vi "Turret Improved.vi"() -> ()   [LabVIEW 2016]
uses:
  <vilib>/Platform/TimedLoop/XDataNode/timing_clust.ctl
  <vilib>/Platform/TimedLoop/XDataNode/nitl_modes.ctl
  <vilib>/Platform/TimedLoop/XDataNode/wakeup.ctl
  TurretStates.ctl
  Drive Commands.ctl
  <vilib>/Analysis/coordinate.llb/Angle Units.ctl
  <vilib>/Analysis/coordinate.llb/Angle Range (Degree).ctl
  <vilib>/Analysis/coordinate.llb/Wrap Angle (scalar).vi
  <vilib>/platform/TimedLoop/XDataNode/XDataNode.xnode
  <vilib>/Platform/TimedLoop/XDataNode/XDNodeRunTimeDep.lvlib
  <vilib>/Analysis/NI_AAL_Angle.lvlib
panel:
  in  "Feed CW":dbl=0.02
  in  "FeedCCW":dbl=-0.02
  in  "Tab Control":T1(tab)
  in  "Min Rate":dbl=0.2
  in  "Lost Target Time?":dbl(knob)=0.5301133241962713 scale=0.0..1.0
  in  "Wait Time in Search":dbl(knob)=0.3769951386039123 scale=0.0..1.0
  in  "Period (ms)":dbl=100.0
  in  "Duty Cycle (%)":dbl=10.0
  in  "Target Range Gains":T2={"proportional gain (Kc)"=0.01, "integral time (Ti, min)"=0.005, "derivative time (Td, min)"=0.0} {"derivative time (Td, min)" format="%.4f"; "integral time (Ti, min)" format="%.8f"; "proportional gain (Kc)" format="%.8f"}
  in  "Target range":cluster{"output high":dbl, "output low":dbl}={"output high"=0.9, "output low"=-0.9}
  in  "Setpoint Tol":dbl=1.0
  in  "Search Gains":T2={"proportional gain (Kc)"=0.018, "integral time (Ti, min)"=0.003, "derivative time (Td, min)"=0.005}
  in  "Search Range":cluster{"output high":dbl, "output low":dbl}={"output high"=0.25, "output low"=-0.25}
  in  "Search Tol":dbl=10.0
  in  "Softstop":dbl=15.0
  in  "Jump to Desired Angle":T2={"proportional gain (Kc)"=0.0155, "integral time (Ti, min)"=0.003, "derivative time (Td, min)"=0.0}
  in  "Jump Output":cluster{"output high":dbl, "output low":dbl}={"output high"=0.5, "output low"=-0.5}
  in  "Valid Target Time Guess":dbl(knob)=0.19161068264500253 scale=0.0..1.0
  in  "Switch outer bound delta":dbl=20.0
  in  "Stable Movemt":dbl(knob)=0.11807450406305693 scale=0.0..1.0
  in  "Guess State Time?":u32
  out "TurretLate?":bool
  in  "Turret Max Speed":dbl(knob)=0.34982498966729664 scale=0.0..1.0
  in  "Reinitalize?":bool
  in  "Range for I":dbl=15.0
  out "Turret":cluster{"Double":dbl, "desired Angle":dbl}(graph)={"Double"=109.84640759396413, "desired Angle"=110.88007694880284}
  out "Motor Output":dbl=0.031700587068503525
  out "Turret State":dbl(graph)
  in  "Test LEDS":bool
  in  "CW Bound":dbl=130.0
  in  "CCW Bound":dbl=-90.0 format="%#_13g"
  in  "Turret Period":i64=20
  out "Turret Duration":i64
  out "Auto Target Lock":bool=TRUE
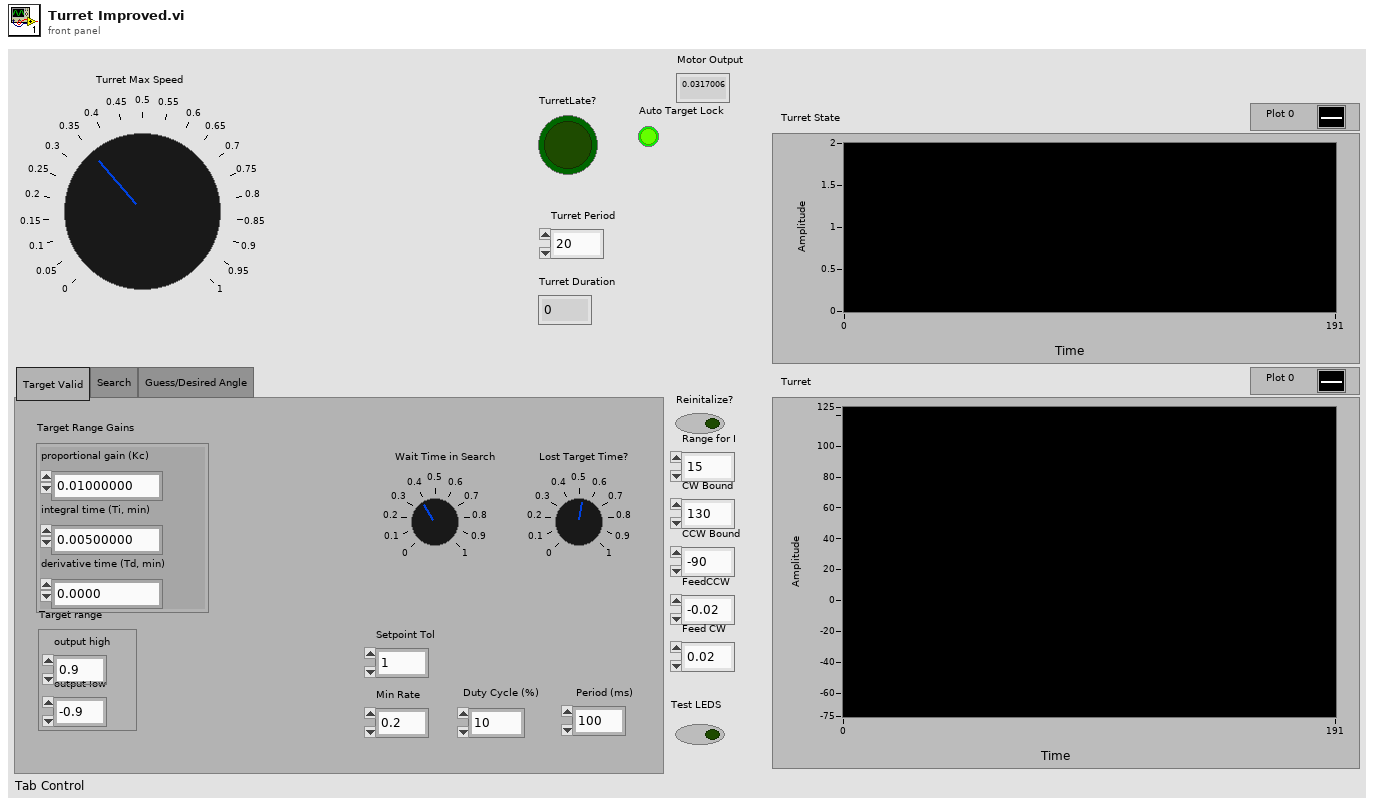
[diagram p1: front panel]
types:
  T1 = enum32{"Target Valid", "Search", "Guess/Desired Angle"}
  T2 = cluster{"proportional gain (Kc)":dbl, "integral time (Ti, min)":dbl, "derivative time (Td, min)":dbl}
  T3 = typedef "TurretStates.ctl" = enum16{"Target Valid in Range", "Guess", "Search", "Desired Angle Shot", "Manual"}
  T4 = typedef "XDNodeRunTimeDep.lvlib/timing_clust.ctl" = cluster{"Expected End [f-1]":u64, "Actual End [f-1]":u64, "Finished Late? [f-1]":bool, "Expected End [i-1]":u64, "Actual End [i-1]":u64, "Finished Late? [i-1]":bool, "Expected Start [i]":u64, "Actual Start [i]":u64, "Expected Start [f]":u64, "Actual Start [f]":u64, "Source Name":string, "Structure Name":string, "Period":i64, "Deadline":i64, "Offset":i64, "Start":i64, "Priority":i32, "Timeout":i32, "Mode":T5, "Wakeup Reason":T6, "Error":errorcluster, "Source Type":string, "Secondary Source Type":string, "Global End Time":u64, "Global Start Time":u64, "Frame Duration":u64, "Iteration Duration":u64, "Assigned CPU":i32, "I/O Scan Engine Mode":u32}
  T5 = typedef "XDNodeRunTimeDep.lvlib/nitl_modes.ctl" = enum32{"No Change", "Process missed periods, maintain original phase", "Discard missed periods, maintain original phase", "Process missed periods, ignore original phase", "Discard missed periods, ignore original phase"}
  T6 = typedef "XDNodeRunTimeDep.lvlib/wakeup.ctl" = enum32{"Normal", "Aborted", "Asynchronous wakeup", "Timing source error", "Timed loop error", "Timeout"}
  T7 = cluster{"Search Gains":cluster{"proportional gain (Kc)":dbl, "integral time (Ti, min)":dbl, "derivative time (Td, min)":dbl}, "Search Range":cluster{"output high":dbl, "output low":dbl}}
  T8 = cluster{"Jump to Desired Angle":cluster{"proportional gain (Kc)":dbl, "integral time (Ti, min)":dbl, "derivative time (Td, min)":dbl}, "Jump Output":cluster{"output high":dbl, "output low":dbl}}
  T9 = cluster{"Target Range Gains":cluster{"proportional gain (Kc)":dbl, "integral time (Ti, min)":dbl, "derivative time (Td, min)":dbl}, "Target range":cluster{"output high":dbl, "output low":dbl}}
  T10 = cluster{"Target Range Gains":cluster{"proportional gain (Kc)":dbl, "integral time (Ti, min)":dbl, "derivative time (Td, min)":dbl}, "Target range":cluster{"output high":dbl, "output low":dbl}}[]
  T11 = typedef "WPI_MotorControlDeviceRef.ctl" = cluster{"DeviceStatus":errorcluster, "Type":T12, "PWM":cluster{"PWM Channel":T13, "DeadBand":T14}, "CAN":cluster{"Device Number":u8, "SetOutput VI Ref":variant, "GetOutput VI Ref":variant, "Enable VI Ref":variant, "Disable VI Ref":variant, "Data":variant}, "Invert":bool}
  T12 = typedef "WPI_MotorControlType.ctl" = enum16{"PWM", "CAN"}
  T13 = typedef "FPGA_DIOPWMChannel.ctl" = enum8{"PWM 0", "PWM 1", "PWM 2", "PWM 3", "PWM 4", "PWM 5", "PWM 6", "PWM 7", "PWM 8", "PWM 9", "PWM MXP 0", "PWM MXP 1", "PWM MXP 2", "PWM MXP 3", "PWM MXP 4", "PWM MXP 5", "PWM MXP 6", "PWM MXP 7", "PWM MXP 8", "PWM MXP 9", "Invalid"}
  T14 = typedef "WPI_PWMDeadband.ctl" = cluster{"Name":string, "maxPositivePwm":i32, "minPositivePwm":i32, "centerPwm":i32, "maxNegativePwm":i32, "minNegativePwm":i32, "angularRange":u16}
  T15 = typedef "Drive Commands.ctl" = enum16{"Manual", "Get Gear", "Score Gear", "Align Rope", "Turn To Angle"}
  T16 = enum8{"setop", "setcolor", "default", "pilot", "ball", "gear", "both", "gearDeliver", "timeWarn", "targeting", "rave", "debug", "Set Power"}
  T17 = typedef "NI_AAL_Angle.lvlib/Angle Range (Degree).ctl" = u16
  T18 = typedef "NI_AAL_Angle.lvlib/Angle Units.ctl" = i32
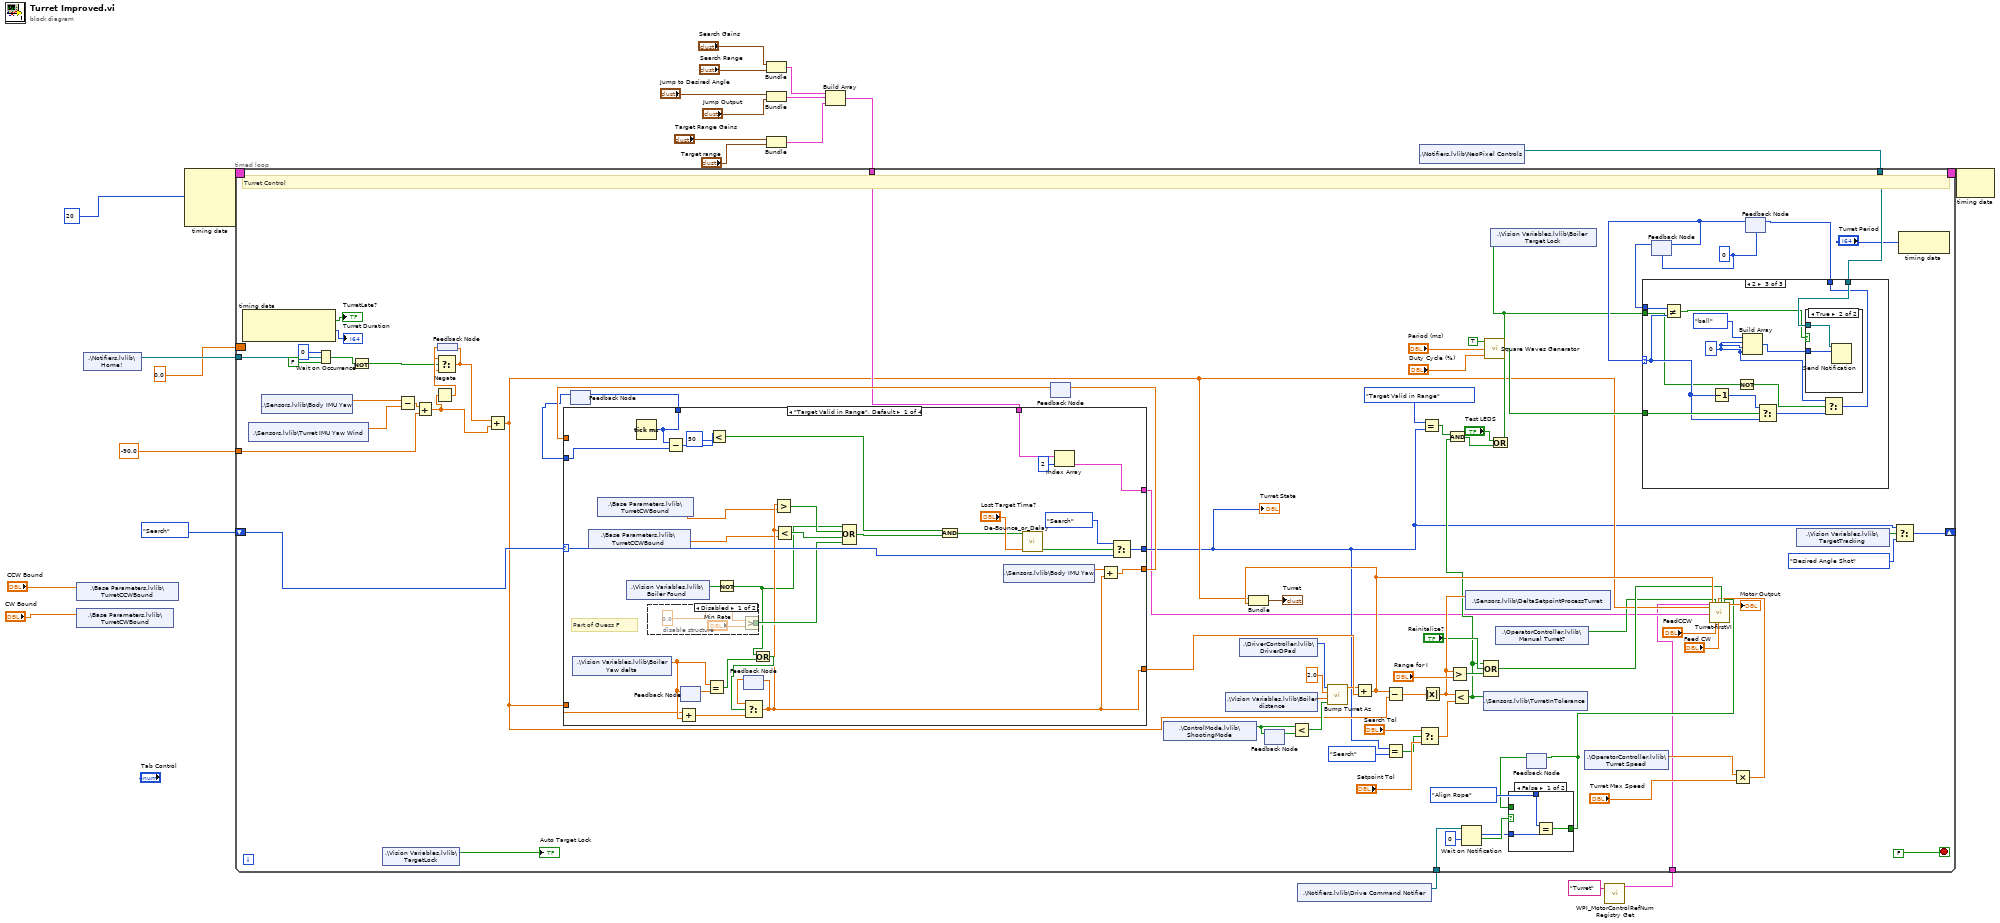
[diagram p0: block diagram]
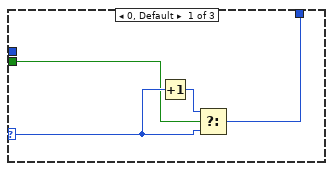
[diagram p3: hidden frame]
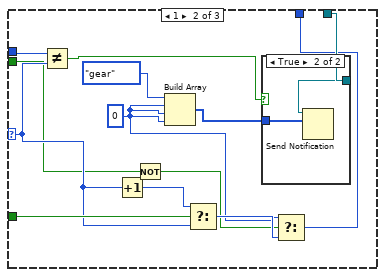
[diagram p4: hidden frame]
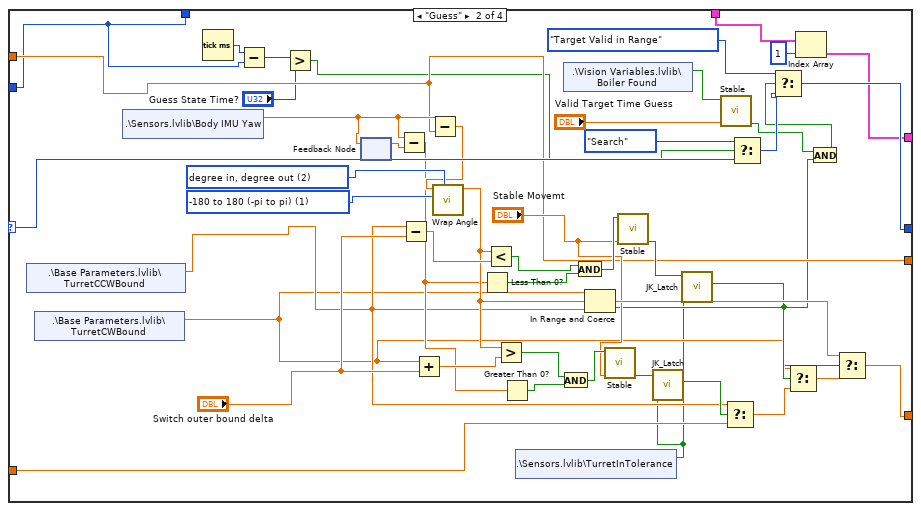
[diagram p8: hidden frame]
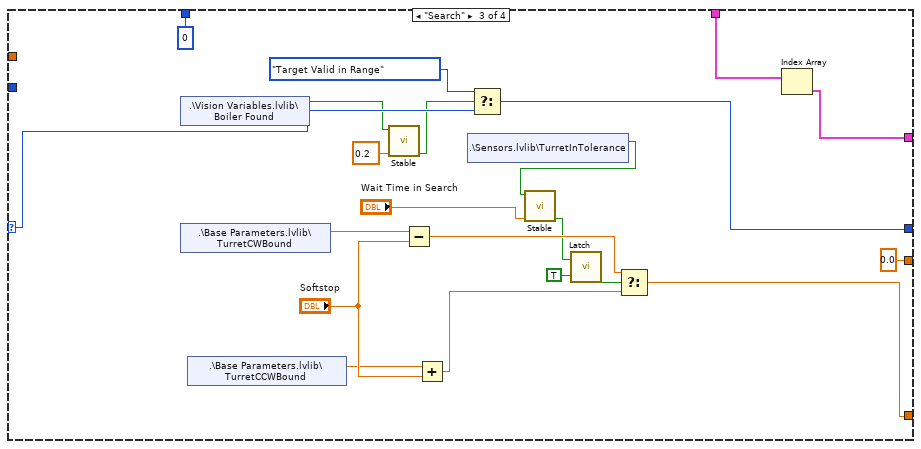
[diagram p9: hidden frame]
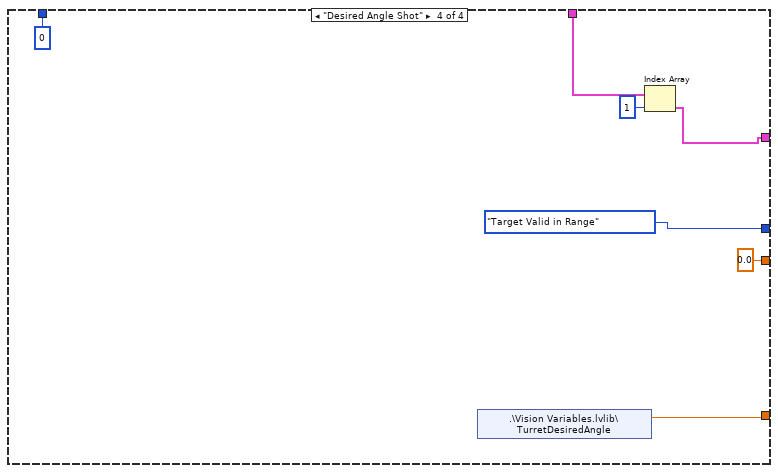
[diagram p10: hidden frame]
diagram:
  n1 = shared-variable ".\\Base Parameters.lvlib\\TurretCCWBound"("CCW Bound") -> ()  [unwired: 1 in, 1 out]
  n2 = shared-variable ".\\Base Parameters.lvlib\\TurretCWBound"("CW Bound") -> ()  [unwired: 1 in, 1 out]
  n3 = shared-variable ".\\Notifiers.lvlib\\Home!"() -> (w17:refnum<k4>)  [unwired: 1 in, 1 out]
  n4 = node-c288(i64 20 ("Period")) -> (w23:T4)  [unwired: 3 in]
  n5 = Bundle("Search Gains"="Search Gains", "Search Range"="Search Range") -> (w11:T7)  [unwired: 1 in]
  n6 = Bundle("Jump to Desired Angle"="Jump to Desired Angle", "Jump Output"="Jump Output") -> (w12:T8)  [unwired: 1 in]
  n7 = Bundle("Target Range Gains"="Target Range Gains", "Target range"="Target range") -> (w13:T9)  [unwired: 1 in]
  n8 = Build Array(w11, w12, w13) -> (w4:T10)
  n9 = shared-variable ".\\Notifiers.lvlib\\Drive Command Notifier"() -> (w3:refnum<notifier>)  [unwired: 1 in, 1 out]
  n10 = shared-variable ".\\Notifiers.lvlib\\NeoPixel Controls"() -> (w19:refnum<notifier>)  [unwired: 1 in, 1 out]
  n11 = call <vilib>:"WPI_MotorControlRefNum Registry Get.vi"("refnum name"="Turret") -> ("MotorControlDevRef"=w1:T11)  [unwired: 9 in, 1 out]
  n12 = timed-loop {
    timing: w23 -> [_]
    timing-out: [_] -> w22
    shift-right: [w58] -> _
    shift-left: TurretStates."Search" -> [w55]
    tunnel: w19 -> [w90]
    tunnel: -90.0 -> [w76]
    tunnel: w17 -> [w74]
    border: 0.0 -> [_]
    tunnel: w4 -> [w39]
    tunnel: w3 -> [w28]
    tunnel: w1 -> [w24]
    stop <- FALSE stop-if-true
    w83 = 0
    # "Turret Control"
    n13 = node-c288() -> (→"TurretLate?":bool, →"Turret Duration":i64)  [unwired: 1 in]
    n14 = shared-variable ".\\Sensors.lvlib\\Turret IMU Yaw Wind"() -> (w103:dbl)  [unwired: 1 in, 1 out]
    n15 = shared-variable ".\\Sensors.lvlib\\Body IMU Yaw"() -> (w102:dbl)  [unwired: 1 in, 1 out]
    n16 = Wait on Occurrence(1:FALSE ("ignore previous (T)"), 2:w74, 3:0 ("ms timeout (-1)")) -> (0:w72:bool)
    n17 = Not(x=w72) -> (.not. x?=w61:bool)
    n18 = shared-variable ".\\Vision Variables.lvlib\\TargetLock"() -> (→"Auto Target Lock":bool)  [unwired: 1 in, 1 out]
    n19 = Subtract(x=w102, y=w103) -> (x-y=w75:dbl)
    n20 = Add(x=w75, y=w76) -> (x+y=w63:dbl)
    n21 = Negate(x=w63) -> (-x=w65:dbl)
    n22 = feedback #1() -> (w64:dbl)
    n23 = Select(t=w65, s=w61, f=w64) -> (s? t:f=w62:dbl)
    n24 = feedback-in #1(w62) -> ()
    n25 = Add(x=w62, y=w63) -> (x+y=w36:dbl)
    n26 = feedback #2() -> (w92:u32)  [unwired: 1 in]
    n27 = feedback #3() -> (w97:dbl)  [unwired: 1 in]
    n28 = case shown="\"Target Valid in Range\", Default" w55 {
      selector: w55 -> [w169 w222 w243 _]
      tunnel: w36 -> [w164 w218 _ _]
      tunnel: [w148 w194 w245 TurretStates."Target Valid in Range"] -> w34
      tunnel: [w152 w215 w239 w250] -> w54
      tunnel: w97 -> [_ w196 _ _]
      tunnel: [w151 w196 0.0 ("Double") 0.0 ("Double")] -> w91
      tunnel: [w162 w187 u32 0 ("millisecond timer value") u32 0 ("millisecond timer value")] -> w93
      tunnel: w92 -> [w161 w187 _ _]
      tunnel: [w144 w178 w225 w247] -> w25
      tunnel: w39 -> [w143 w180 w226 w248]
      frame "Target Valid in Range", Default {
        # "Part of Guess F"
        n29 = shared-variable ".\\Vision Variables.lvlib\\Boiler Yaw delta"() -> (w173:dbl)  [unwired: 1 in, 1 out]
        n30 = shared-variable ".\\Base Parameters.lvlib\\TurretCCWBound"() -> (w147:dbl)  [unwired: 1 in, 1 out]
        n31 = shared-variable ".\\Base Parameters.lvlib\\TurretCWBound"() -> (w146:dbl)  [unwired: 1 in, 1 out]
        n32 = shared-variable ".\\Vision Variables.lvlib\\Boiler Found"() -> (w170:bool)  [unwired: 1 in, 1 out]
        n33 = Tick Count (ms)() -> (millisecond timer value=w162:u32)
        n34 = disable-structure shown="Disabled" {
          disable-tunnel: [w176 _] -> w163
          frame Disabled {
            n35 = Greater?(x=0.0, y="Min Rate") -> (0:w176:bool)
          }
          frame Enabled {
          }
        }
        n36 = Subtract(x=w162, y=w161) -> (x-y=w160:u32)
        n37 = Add(x=w164, y=w173) -> (x+y=w172:dbl)
        n38 = feedback-in #4(w173) -> ()
        n39 = feedback #4() -> (w174:dbl)  [unwired: 1 in]
        n40 = Equal?(x=w173, y=w174) -> (x = y?=w155:bool)
        n41 = Less?(x=w160, y=u32 50) -> (x < y?=w158:bool)
        n42 = Not(x=w170) -> (.not. x?=w150:bool)
        n43 = feedback #5() -> (w171:dbl)  [unwired: 1 in]
        n44 = Or(x=w150, y=w155) -> (x .or. y?=w154:bool)
        n45 = Select(t=w171, s=w154, f=w172) -> (s? t:f=w152:dbl)
        n46 = feedback-in #5(w152) -> ()
        n47 = Greater?(x=w152, y=w146) -> (0:w166:bool)
        n48 = Less?(x=w152, y=w147) -> (x < y?=w165:bool)
        n49 = Compound Arithmetic op=OR(w150, w166, w165, w163) -> (w157:bool)
        n50 = And(x=w158, y=w157) -> (x .and. y?=w156:bool)
        n51 = shared-variable ".\\Sensors.lvlib\\Body IMU Yaw"() -> (w153:dbl)  [unwired: 1 in, 1 out]
        n52 = call <userlib>:"De-Bounce_or_Delay.vi"("Eval Period (sec)"="Lost Target Time?", "Signal Input"=w156) -> ("Stable"=w149:bool)  [unwired: 9 in]
        n53 = Index Array(array=w143, index=2) -> (element=w144:T9)
        n54 = Add(x=w153, y=w152) -> (x+y=w151:dbl)
        n55 = Select(t=TurretStates."Search", s=w149, f=w169) -> (s? t:f=w148:T3)
      }
      frame "Guess" {
        w213 = T17 1 items=["none", "-180 to 180 (-pi to pi)", "0 to 360 (0 to 2pi)"] ("angle range")
        w214 = T18 2 items=["radian in, radian out", "radian in, degree out", "degree in, degree out", "degree in, radian out"] ("angle units")
        n56 = shared-variable ".\\Base Parameters.lvlib\\TurretCCWBound"() -> (w183:dbl)  [unwired: 1 in, 1 out]
        n57 = shared-variable ".\\Base Parameters.lvlib\\TurretCWBound"() -> (w182:dbl)  [unwired: 1 in, 1 out]
        n58 = shared-variable ".\\Sensors.lvlib\\Body IMU Yaw"() -> (w208:dbl)  [unwired: 1 in, 1 out]
        n59 = Tick Count (ms)() -> (millisecond timer value=w188:u32)
        n60 = Subtract(x=w188, y=w187) -> (x-y=w186:u32)
        n61 = Greater?(x=w186, y="Guess State Time?") -> (0:w184:bool)
        n62 = feedback-in #6(w208) -> ()
        n63 = feedback #6() -> (w209:dbl)  [unwired: 1 in]
        n64 = Subtract(x=w208, y=w209) -> (x-y=w202:dbl)
        n65 = Subtract(x=w183, y="Switch outer bound delta") -> (x-y=w220:dbl)
        n66 = Add(x=w182, y="Switch outer bound delta") -> (x+y=w219:dbl)
        n67 = Subtract(x=w208, y=w196) -> (x-y=w212:dbl)
        n68 = call-poly <vilib>:"Wrap Angle.vi"("angle units"=w214, "angle range"=w213, "angle in"=w212) -> ("angle out"=w211:dbl)  [unwired: 7 in, 1 out]
        n69 = Less Than 0?(x=w202) -> (x < 0?=w205:bool)
        n70 = Less?(x=w211, y=w220) -> (x < y?=w206:bool)
        n71 = Greater?(x=w211, y=w219) -> (0:w210:bool)
        n72 = Greater Than 0?(x=w202) -> (x > 0?=w207:bool)
        n73 = shared-variable ".\\Sensors.lvlib\\TurretInTolerance"() -> (w181:bool)  [unwired: 1 in, 1 out]
        n74 = And(x=w210, y=w207) -> (x .and. y?=w199:bool)
        n75 = shared-variable ".\\Vision Variables.lvlib\\Boiler Found"() -> (w193:bool)  [unwired: 1 in, 1 out]
        n76 = And(x=w206, y=w205) -> (x .and. y?=w201:bool)
        n77 = In Range and Coerce(upper limit=w182, x=w211, lower limit=w183) -> (In Range?=w189:bool)  [unwired: 1 out]
        n78 = call <userlib>:"Stable.vi"("Eval Period (sec)"="Stable Movemt", "Signal Input"=w199) -> ("Stable"=w198:bool)  [unwired: 9 in]
        n79 = call <userlib>:"Stable.vi"("Eval Period (sec)"="Stable Movemt", "Signal Input"=w201) -> ("Stable"=w200:bool)  [unwired: 9 in]
        n80 = call <userlib>:"JK_Latch.vi"("Reset"=w181, "Set"=w198) -> ("Q"=w204:bool)  [unwired: 5 in]
        n81 = call <userlib>:"JK_Latch.vi"("Reset"=w181, "Set"=w200) -> ("Q"=w203:bool)  [unwired: 5 in]
        n82 = call <userlib>:"Stable.vi"("Eval Period (sec)"="Valid Target Time Guess", "Signal Input"=w193) -> ("Stable"=w191:bool)  [unwired: 9 in]
        n83 = Select(t=w183, s=w204, f=w218) -> (s? t:f=w217:dbl)
        n84 = Select(t=TurretStates."Search", s=w184, f=w222) -> (s? t:f=w195:T3)
        n85 = Select(t=w182, s=w203, f=w217) -> (s? t:f=w216:dbl)
        n86 = Index Array(array=w180, index=1) -> (element=w178:T9)
        n87 = And(x=w191, y=w189) -> (x .and. y?=w190:bool)
        n88 = Select(t=TurretStates."Target Valid in Range", s=w190, f=w195) -> (s? t:f=w194:T3)
        n89 = Select(t=w211, s=w189, f=w216) -> (s? t:f=w215:dbl)
      }
      frame "Search" {
        n90 = shared-variable ".\\Vision Variables.lvlib\\Boiler Found"() -> (w234:bool)  [unwired: 1 in, 1 out]
        n91 = shared-variable ".\\Base Parameters.lvlib\\TurretCWBound"() -> (w228:dbl)  [unwired: 1 in, 1 out]
        n92 = shared-variable ".\\Base Parameters.lvlib\\TurretCCWBound"() -> (w229:dbl)  [unwired: 1 in, 1 out]
        n93 = call <userlib>:"Stable.vi"("Eval Period (sec)"=0.2, "Signal Input"=w234) -> ("Stable"=w233:bool)  [unwired: 9 in]
        n94 = Subtract(x=w228, y="Softstop") -> (x-y=w241:dbl)
        n95 = Add(x=w229, y="Softstop") -> (x+y=w240:dbl)
        n96 = shared-variable ".\\Sensors.lvlib\\TurretInTolerance"() -> (w227:bool)  [unwired: 1 in, 1 out]
        n97 = Select(t=TurretStates."Target Valid in Range", s=w233, f=w243) -> (s? t:f=w245:T3)
        n98 = call <userlib>:"Stable.vi"("Eval Period (sec)"="Wait Time in Search", "Signal Input"=w227) -> ("Stable"=w230:bool)  [unwired: 9 in]
        n99 = call <userlib>:"Latch.vi"("Edge"=TRUE ("Edge:  When lit the output is \"True\" for this control"), "In"=w230) -> ("Out"=w235:bool)
        n100 = Select(t=w241, s=w235, f=w240) -> (s? t:f=w239:dbl)
        n101 = Index Array(array=w226) -> (element=w225:T9)  [unwired: 1 in]
      }
      frame "Desired Angle Shot" {
        n102 = shared-variable ".\\Vision Variables.lvlib\\TurretDesiredAngle"() -> (w250:dbl)  [unwired: 1 in, 1 out]
        n103 = Index Array(array=w248, index=1) -> (element=w247:T9)
      }
    }
    "Turret State" <- w34
    n104 = feedback-in #2(w93) -> ()
    n105 = feedback-in #3(w91) -> ()
    n106 = shared-variable ".\\ControlMode.lvlib\\ShootingMode"() -> (w48:bool)  [unwired: 1 in, 1 out]
    n107 = shared-variable ".\\Vision Variables.lvlib\\Boiler distance"() -> (w50:dbl)  [unwired: 1 in, 1 out]
    n108 = shared-variable ".\\DriverController.lvlib\\DriverDPad"() -> (w49:i16)  [unwired: 1 in, 1 out]
    n109 = feedback #7() -> (w47:bool)  [unwired: 1 in]
    n110 = feedback-in #7(w48) -> ()
    n111 = Less?(x=w48, y=w47) -> (x < y?=w46:bool)
    n112 = call "Bump Turret Az.vi"("reset"=w46, "D"=w50, "d"=2.0, "D-Pad"=w49) -> ("offset"=w52:dbl)  [unwired: 7 in]
    n113 = Add(x=w52, y=w54) -> (x+y=w53:dbl)
    n114 = Bundle(w36, w53) -> (→"Turret":cluster{dbl, dbl})  [unwired: 1 in]
    n115 = Subtract(x=w53, y=w36) -> (x-y=w98:dbl)
    n116 = Equal?(x=w34, y=TurretStates."Search") -> (x = y?=w40:bool)
    n117 = Select(t="Search Tol", s=w40, f="Setpoint Tol") -> (s? t:f=w42:dbl)
    n118 = Equal?(x=TurretStates."Target Valid in Range", y=w34) -> (x = y?=w80:bool)
    n119 = Absolute Value(x=w98) -> (abs(x)=w67:dbl)
    n120 = Greater?(x=w67, y="Range for I") -> (0:w56:bool)
    n121 = Less?(x=w67, y=w42) -> (x < y?=w45:bool)
    n122 = And(x=w80, y=w45) -> (x .and. y?=w79:bool)
    n123 = Wait on Notification(notifier=w28, timeout in ms (-1)=0) -> (notification=w31:T15, timed out?=w32:bool)  [unwired: 2 in, 2 out]
    n124 = shared-variable ".\\Sensors.lvlib\\DeltaSetpointProcessTurret"(w67) -> ()  [unwired: 1 in, 1 out]
    n125 = Compound Arithmetic op=OR(w45, "Reinitalize?", w56) -> (w37:bool)
    n126 = shared-variable ".\\Sensors.lvlib\\TurretInTolerance"(w45) -> ()  [unwired: 1 in, 1 out]
    n127 = call "Square Waves Generator.vi"("Duty Cycle (%)"="Duty Cycle (%)", "Period (ms)"="Period (ms)", "Enable"=TRUE) -> ("Signal"=w85:bool)
    n128 = Or(x="Test LEDS", y=w79) -> (x .or. y?=w78:bool)
    n129 = shared-variable ".\\Vision Variables.lvlib\\Boiler Target Lock"(w78) -> ()  [unwired: 1 in, 1 out]
    n130 = shared-variable ".\\OperatorController.lvlib\\Manual Turret?"() -> (w35:bool)  [unwired: 1 in, 1 out]
    n131 = feedback #8() -> (w29:bool)  [unwired: 1 in]
    n132 = case shown="False" w32 {
      tunnel: w31 -> [w107 _]
      tunnel: Drive_Commands."Align Rope" ("notification") -> [w106 _]
      tunnel: [w105 w108] -> w27
      tunnel: w29 -> [_ w108]
      frame False {
        n133 = Equal?(x=w106, y=w107) -> (x = y?=w105:bool)
      }
      frame True {
      }
    }
    n134 = feedback-in #8(w27) -> ()
    n135 = shared-variable ".\\OperatorController.lvlib\\Turret Speed"() -> (w68:dbl)  [unwired: 1 in, 1 out]
    n136 = feedback #9(w83) -> (w82:i32)
    n137 = Multiply(x=w68, y="Turret Max Speed") -> (x*y=w26:dbl)
    n138 = call "Turret-firstVI.vi"("MotorControlDevRef"=w24, "Current angle"=w36, "desired Angle"=w53, "PID Values"=w25, "Manual"=w35, "Feed CCW"="FeedCCW", "Output"=w26, "Feed CW"="Feed CW", "reinitialize? (F)"=w37, "Climbing?"=w27) -> ("Motor Output"=→"Motor Output":dbl)  [unwired: 9 in]
    n139 = feedback #10(w83) -> (w84:i32)
    n140 = case shown="2" w84 {
      selector: w84 -> [w110 w118 w133]
      tunnel: w90 -> [_ w125 w140]
      tunnel: [w112 w114 w129] -> w89
      tunnel: w85 -> [_ w122 w137]
      tunnel: w82 -> [_ w120 w135]
      tunnel: w78 -> [w109 w117 w132]
      frame 0, Default {
        n141 = Increment(x=w110) -> (x+1=w111:i32)
        n142 = Select(t=w111, s=w109, f=w110) -> (s? t:f=w112:i32)
      }
      frame 1 {
        w115 = 0
        n143 = Not Equal?(x=w120, y=w118) -> (x != y?=w119:bool)
        n144 = Increment(x=w118) -> (x+1=w121:i32)
        n145 = Not(x=w117) -> (.not. x?=w113:bool)
        n146 = Build Array(T16."gear" ("Enum"), w115, w115, w115) -> (w123:i32[])
        n147 = Select(t=w121, s=w122, f=w118) -> (s? t:f=w116:i32)
        n148 = case shown="True" w119 {
          tunnel: w125 -> [_ w127]
          tunnel: w123 -> [_ w126]
          frame False {
          }
          frame True {
            n149 = Send Notification(notification=w126, notifier=w127) -> ()  [unwired: 1 in, 2 out]
          }
        }
        n150 = Select(t=w115, s=w113, f=w116) -> (s? t:f=w114:i32)
      }
      frame 2 {
        w130 = 0
        n151 = Not Equal?(x=w135, y=w133) -> (x != y?=w134:bool)
        n152 = Decrement(x=w133) -> (x-1=w136:i32)
        n153 = Not(x=w132) -> (.not. x?=w128:bool)
        n154 = Build Array(T16."ball" ("Enum"), w130, w130, w130) -> (w138:i32[])
        n155 = Select(t=w136, s=w137, f=w133) -> (s? t:f=w131:i32)
        n156 = case shown="True" w134 {
          tunnel: w140 -> [_ w142]
          tunnel: w138 -> [_ w141]
          frame False {
          }
          frame True {
            n157 = Send Notification(notification=w141, notifier=w142) -> ()  [unwired: 1 in, 2 out]
          }
        }
        n158 = Select(t=w130, s=w128, f=w131) -> (s? t:f=w129:i32)
      }
    }
    n159 = feedback-in #9(w84) -> ()
    n160 = feedback-in #10(w89) -> ()
    n161 = shared-variable ".\\Vision Variables.lvlib\\TargetTracking"() -> (w60:bool)  [unwired: 1 in, 1 out]
    n162 = Select(t=w34, s=w60, f=TurretStates."Desired Angle Shot" ("x")) -> (s? t:f=w58:T3)
    n163 = node-c288("Turret Period") -> ()  [unwired: 1 out]
  }
  n164 = node-c288(w22) -> ()  [unwired: 1 out]
